vi "set_moving_by_name.vi"(8 "error in (no error)":errorcluster caption="错误输入（无错误）", 9 "moving?":bool, 10 "name":string, 11 "MotorSystem输入":refnum<class "MotorSystem.lvclass">) -> (0 "error out":errorcluster caption="错误输出", 3 "MotorSystem输出":refnum<class "MotorSystem.lvclass">)   [LabVIEW 2016, in "MotionControl.lvlib" / "MotorSystem.lvclass"]
uses:
  <userlib>/MotionControl/MotorSystem/MotorSystem.lvclass
  <userlib>/MotionControl/MotorSystem/MotorSystem.lvclass/MotorSystem.ctl
  <userlib>/MotionControl/OneMotion/OneMotion.lvclass/OneMotion.ctl
  <userlib>/MotionControl/StepMotor/StepMotor.lvclass/StepMotor.ctl
  <userlib>/MotionControl/StepMotor/StepMotor.lvclass
  <userlib>/MotionControl/OneMotion/OneMotion.lvclass
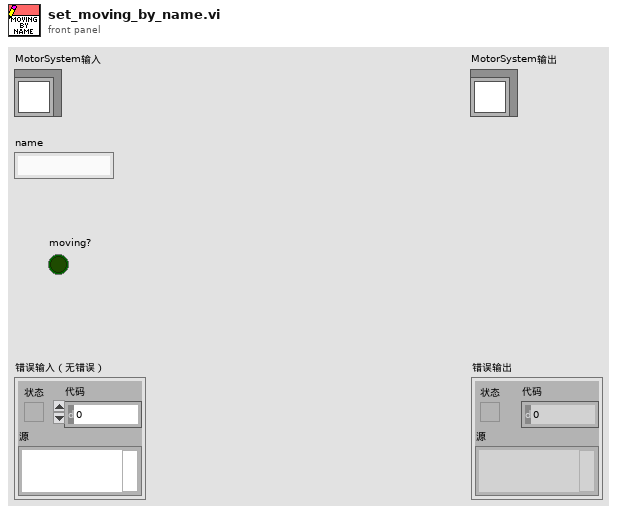
[diagram p1: front panel]
types:
  T1 = typedef "MotionControl.lvlib/MotorSystem.lvclass/MotionCluster.ctl" = cluster{"OneMotion.lvclass":refnum<class "OneMotion.lvclass">, "connected?":bool, "default enabled?":bool, "enabled?":bool}
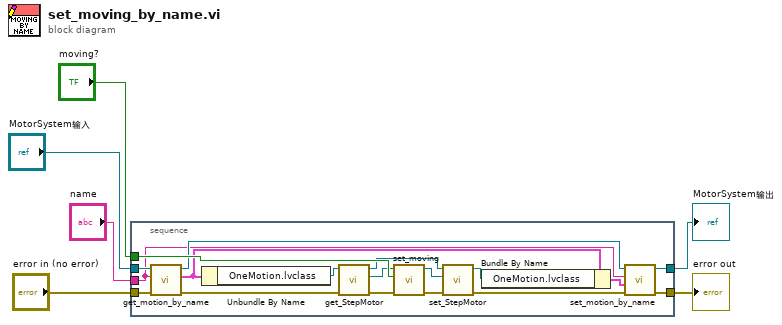
[diagram p0: block diagram]
diagram:
  n1 = stacked-sequence {
    tunnel: [w7] -> w6
    tunnel: [w13] -> w4
    tunnel: "MotorSystem输入" -> [w24]
    tunnel: "name" -> [w14]
    tunnel: "moving?" -> [w23]
    tunnel: "error in (no error)" -> [w12]
    frame #0 {
      n2 = call <userlib>:"get_motion_by_name.vi"("error in (no error)"=w12, "name"=w14, "MotorSystem in"=w24) -> ("error out"=w11:errorcluster, "motion cluster"=w22:T1, "MotorSystem out"=w16:refnum<class "MotorSystem.lvclass">)  [unwired: 6 in]
      n3 = Unbundle By Name(w22) -> ("OneMotion.lvclass"=w21:refnum<class "OneMotion.lvclass">)
      n4 = call <userlib>:"get_StepMotor.vi"("error in (no error)"=w11, "OneMotion输入"=w21) -> ("error out"=w10:errorcluster, "StepMotor.lvclass"=w20:refnum<class "StepMotor.lvclass">, "OneMotion输出"=w18:refnum<class "OneMotion.lvclass">)  [unwired: 7 in]
      n5 = call <userlib>:"set_moving.vi"("error in (no error)"=w10, "moving?"=w23, "StepMotor输入"=w20) -> ("error out"=w9:errorcluster, "StepMotor输出"=w19:refnum<class "StepMotor.lvclass">)  [unwired: 7 in]
      n6 = call <userlib>:"set_StepMotor.vi"("error in (no error)"=w9, "StepMotor.lvclass"=w19, "OneMotion输入"=w18) -> ("error out"=w8:errorcluster, "OneMotion输出"=w17:refnum<class "OneMotion.lvclass">)  [unwired: 7 in]
      n7 = Bundle By Name(cluster=w22, "OneMotion.lvclass"=w17) -> (w15:T1)
      n8 = call <userlib>:"set_motion_by_name.vi"("error in (no error)"=w8, "簇"=w15, "name"=w14, "MotorSystem输入"=w16) -> ("error out"=w7:errorcluster, "MotorSystem输出"=w13:refnum<class "MotorSystem.lvclass">)  [unwired: 6 in]
    }
  }
  "error out" <- w6
  "MotorSystem输出" <- w4
